vi "canBePlaced.vi"(7 "array":i32[][](array[numeric]), 10 "index (col)":i32, 11 "index (row)":i32) -> (3 "color":cluster{u32, u32}[](array[cluster]))   [LabVIEW 2022 SP3, in "drawPlate.lvlib"]
uses:
  drawPlate.lvlib
panel:
  # "if (can be placed) \n       display button;"
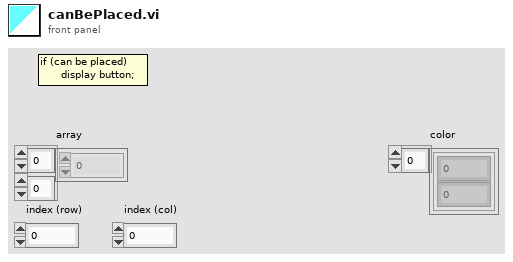
[diagram p1: front panel]
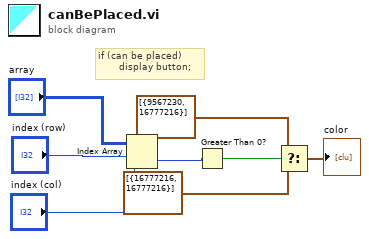
[diagram p0: block diagram]
diagram:
  # "if (can be placed) \n       display button;"
  n1 = Index Array(array="array", index (row)="index (row)", index (col)="index (col)") -> (element=w6:i32)
  n2 = Greater Than 0?(x=w6) -> (x > 0?=w1:bool)
  n3 = Select(t=cluster{u32, u32}[] [{9567230, 16777216}] ("Colors [4]"), s=w1, f=cluster{u32, u32}[] [{16777216, 16777216}] ("Colors [4]")) -> (s? t:f=→"color":cluster{u32, u32}[])
